vi "Open Connection.vi"(8 "error in (no error)":errorcluster, 10 "Connection string":string="server=127.0.0.1;uid=root;pwd=Nitrog3n;database=test", 11 "mysql in":refnum<class "mysql.lvclass">) -> (0 "error out":errorcluster={"status"=TRUE, "code"=1172, "source"="Invoke Node System.Reflection.TargetInvocationException: Exception has been thrown by the target of an invocation.\n\tInner Exception: MySql.Data.MySqlClient.MySqlException: Authentication to host '127.0.0.1' for user 'root' using method 'caching_sha2_password' failed with message: Access denied for user 'root'@'localhost' (using password: YES)\n\tInner Exception: MySql.Data.MySqlClient.MySqlException: Access denied for user 'root'@'localhost' (using password: YES) <append><b>MySql.Data.MySqlClient.MySqlException</b> in mysql.lvlib:mysql.lvclass:Open Connection.vi"}, 3 "mysql out":refnum<class "mysql.lvclass">)   [LabVIEW 2020, in "mysql.lvlib" / "mysql.lvclass"]
uses:
  mysql.lvclass
  MySql.Data
  mysql.lvclass/mysql.ctl
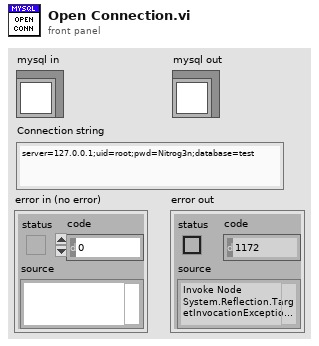
[diagram p1: front panel]
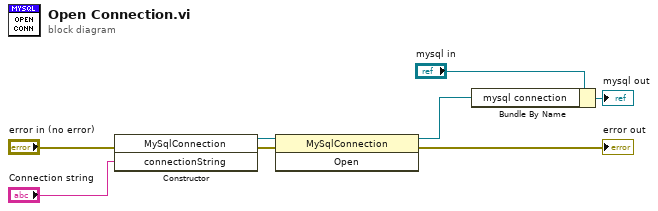
[diagram p0: block diagram]
diagram:
  n1 = constructor class="MySqlConnection"(error in="error in (no error)", "connectionString"="Connection string") -> (reference out=w4:refnum<k24>, error out=w5:errorcluster)  [unwired: 2 in, 2 out]
  n2 = invoke class="MySqlConnection" method="Open"(reference=w4, error in=w5) -> (reference out=w2:refnum<k24>, error out=→"error out":errorcluster)  [unwired: 1 in, 1 out]
  n3 = Bundle By Name(cluster="mysql in", "mysql connection"=w2) -> (→"mysql out":refnum<class "mysql.lvclass">)
